vi "Calculate Fuel AVGs Send Fuel.vi"(8 "error in":errorcluster, 10 "Old Fuel Flows":dbl[][][](array[numeric]), 11 "New Fuel Flows":dbl[][](array[numeric])) -> (0 "error out":errorcluster, 3 "Combined Fuel Flows":dbl[][][](array[numeric]))   [LabVIEW 2017, in "Akwizycja.lvlib"]
uses:
  Akwizycja.lvlib
panel:
  in  "Avg fuel":T1
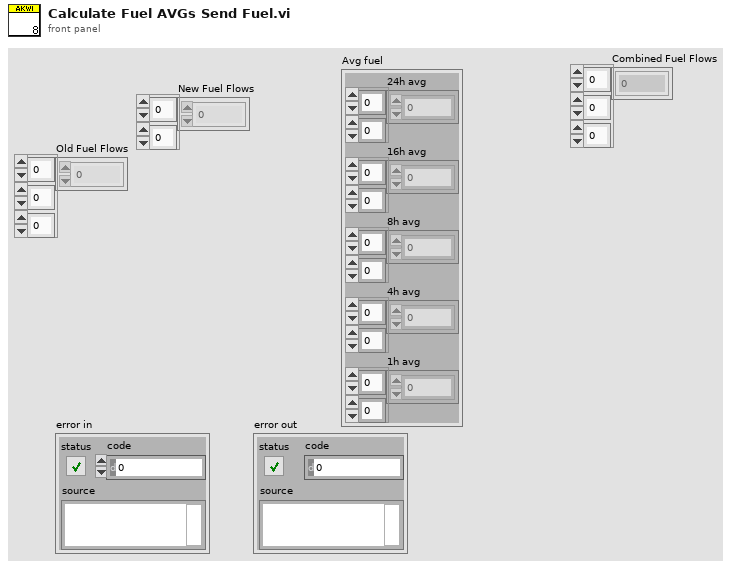
[diagram p1: front panel]
types:
  T1 = cluster{"24h avg":dbl[][], "16h avg":dbl[][], "8h avg":dbl[][], "4h avg":dbl[][], "1h avg":dbl[][]}
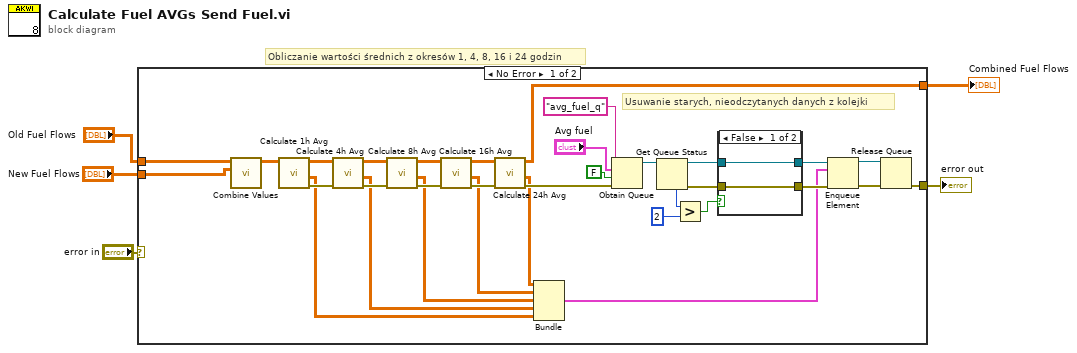
[diagram p0: block diagram]
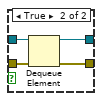
[diagram p2: hidden frame]
diagram:
  # "Obliczanie wartości średnich z okresów 1, 4, 8, 16 i 24 godzin"
  n1 = case shown="No Error" "error in" {
    selector: "error in" -> [_ w46]
    tunnel: [w21 w46] -> w5
    tunnel: "Old Fuel Flows" -> [w9 w45]
    tunnel: "New Fuel Flows" -> [w8 _]
    tunnel: [w7 w45] -> w1
    frame No Error {
      # "Usuwanie starych, nieodczytanych danych z kolejki"
      n2 = call "Combine Values.vi"("New Values"=w8, "Old Values"=w9) -> ("Combined Values"=w10:dbl[][][])  [unwired: 8 in, 1 out]
      n3 = call "Calculate 1h Avg.vi"("Values in"=w10) -> ("error out"=w31:errorcluster, "1h avg"=w27:dbl[][], "Values out"=w35:dbl[][][])  [unwired: 8 in]
      n4 = call "Calculate 4h Avg.vi"("error in"=w31, "Values in"=w35) -> ("error out"=w32:errorcluster, "4h avg"=w28:dbl[][], "Values out"=w36:dbl[][][])  [unwired: 7 in]
      n5 = call "Calculate 8h Avg.vi"("error in"=w32, "Values in"=w36) -> ("error out"=w33:errorcluster, "8h avg"=w29:dbl[][], "Values out"=w37:dbl[][][])  [unwired: 7 in]
      n6 = call "Calculate 16h Avg.vi"("error in (no error)"=w33, "Values in"=w37) -> ("error out"=w34:errorcluster, "16h avg"=w30:dbl[][], "Values out"=w38:dbl[][][])  [unwired: 7 in]
      n7 = call "Calculate 24h Avg.vi"("error in"=w34, "Values in"=w38) -> ("error out"=w24:errorcluster, "24h avg"=w20:dbl[][], "Values out"=w7:dbl[][][])  [unwired: 7 in]
      n8 = Bundle("24h avg"=w20, "16h avg"=w30, "8h avg"=w29, "4h avg"=w28, "1h avg"=w27) -> (w12:T1)  [unwired: 1 in]
      n9 = Obtain Queue(name (unnamed)="avg_fuel_q", element data type="Avg fuel", create if not found? (T)=FALSE, error in (no error)=w24) -> (queue out=w19:refnum<queue>)  [unwired: 1 in, 2 out]
      n10 = Get Queue Status(queue=w19) -> (queue out=w15:refnum<queue>, error out=w18:errorcluster, # elements in queue=w17:i32)  [unwired: 2 in, 5 out]
      n11 = Greater?(x=w17, y=2) -> (0:w11:bool)
      n12 = case shown="False" w11 {
        tunnel: w18 -> [w39 w44]
        tunnel: w15 -> [w40 w43]
        tunnel: [w40 w42] -> w14
        tunnel: [w39 w41] -> w13
        frame False {
        }
        frame True {
          n13 = Dequeue Element(queue=w43, error in (no error)=w44) -> (queue out=w42:refnum<queue>, error out=w41:errorcluster)  [unwired: 1 in, 2 out]
        }
      }
      n14 = Enqueue Element(queue=w14, element=w12, error in (no error)=w13) -> (queue out=w23:refnum<queue>, error out=w22:errorcluster)  [unwired: 1 in, 1 out]
      n15 = Release Queue(queue=w23, error in (no error)=w22) -> (error out=w21:errorcluster)  [unwired: 1 in, 2 out]
    }
    frame Error {
    }
  }
  "error out" <- w5
  "Combined Fuel Flows" <- w1
